vi "saveImage.vi"(8 "error in (no error)":errorcluster, 9 "16bit image data":i16[][](array[numeric]), 10 "Path":path, 11 "Pixelfly in":refnum<class "Pixelfly.lvclass">) -> (0 "error out":errorcluster, 3 "Pixelfly out":refnum<class "Pixelfly.lvclass">)   [LabVIEW 2009]
uses:
  Camera/Camera.lvclass
  Camera/Pixelfly/Pixelfly.lvclass
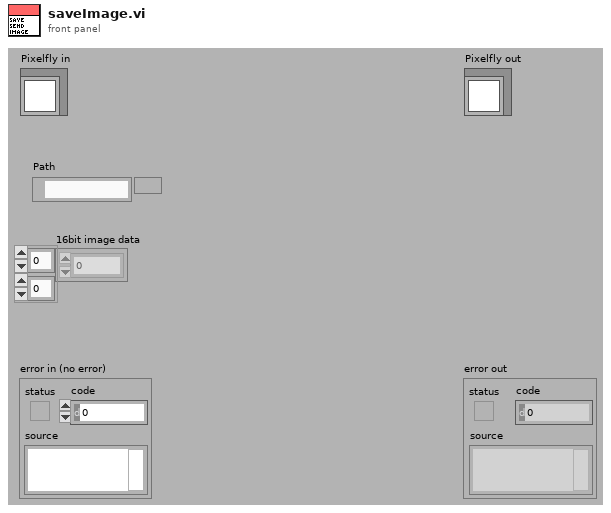
[diagram p1: front panel]
types:
  T1 = typedef "Image Type" = u32
  T2 = typedef "IMAQ Image.ctl" = refnum<image>
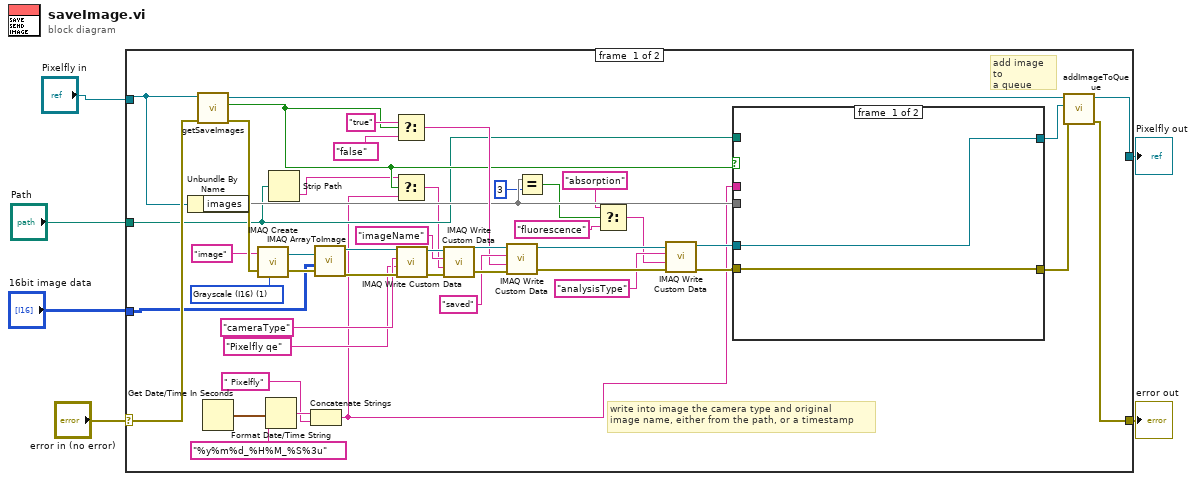
[diagram p0: block diagram]
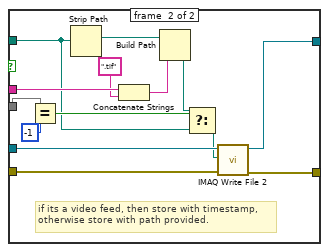
[diagram p2: hidden frame]
diagram:
  n1 = case shown="No Error" "error in (no error)" {
    selector: "error in (no error)" -> [w52 w70]
    tunnel: [w44 w70] -> w5
    tunnel: [w45 w69] -> w3
    tunnel: "Pixelfly in" -> [w25 w69]
    tunnel: "Path" -> [w11 _]
    tunnel: "16bit image data" -> [w7 _]
    frame #0 {
      w49 = T1 1 items=["Grayscale (U8)", "Grayscale (I16)", "Grayscale (SGL)", "Complex (CSG)", "RGB (U32)", "HSL (U32)", "RGB (U64)", "Grayscale (U16)"] ("Image Type")
      # "write into image the camera type and original\nimage name, either from the path, or a timestamp"
      # "add image to\na queue"
      n2 = Unbundle By Name(w25) -> ("images"=w21)
      n3 = call "getSaveImages.vi"("error in (no error)"=w52, "Camera in"=w25) -> ("error out"=w51:errorcluster, "saveImages?"=w12:bool, "Camera out"=w46:refnum<class "Pixelfly.lvclass">)  [unwired: 7 in]
      n4 = Get Date/Time In Seconds() -> (seconds since 1Jan1904=w39:timestamp)
      n5 = call "IMAQ Create"("Image Name"="image", "Image Type"=w49, "error in (no error)"=w51) -> ("New Image"=w48:T2, "error out"=w47:errorcluster)  [unwired: 2 in]
      n6 = Format Date/Time String(time format string (%c)="%y%m%d_%H%M_%S%3u", seconds (now)=w39) -> (date/time string=w37:string)  [unwired: 1 in]
      n7 = Strip Path(path=w11) -> (name=w10:string)  [unwired: 1 out]
      n8 = Concatenate Strings(w37, " Pixelfly") -> (w9:string)
      n9 = call "IMAQ ArrayToImage"("error in (no error)"=w47, "Image Pixels (I16)"=w7, "Image"=w48) -> ("error out"=w42:errorcluster, "Image Out"=w43:T2)  [unwired: 7 in]
      n10 = Select(t="true", s=w12, f="false") -> (s? t:f=w28:string)
      n11 = Select(t=w10, s=w12, f=w9) -> (s? t:f=w8:string)
      n12 = call "IMAQ Write Custom Data"("error in (no error)"=w42, "Custom Data In"="Pixelfly qe", "Key"="cameraType", "Image"=w43) -> ("error out"=w35:errorcluster, "Image Out"=w34:T2)  [unwired: 6 in]
      n13 = call "IMAQ Write Custom Data"("error in (no error)"=w35, "Custom Data In"=w8, "Key"="imageName", "Image"=w34) -> ("error out"=w33:errorcluster, "Image Out"=w32:T2)  [unwired: 6 in]
      n14 = call "IMAQ Write Custom Data"("error in (no error)"=w33, "Custom Data In"=w28, "Key"="saved", "Image"=w32) -> ("error out"=w23:errorcluster, "Image Out"=w24:T2)  [unwired: 6 in]
      n15 = Equal?(x=w21, y=3) -> (x = y?=w19:bool)
      n16 = Select(t="absorption", s=w19, f="fluorescence") -> (s? t:f=w16:string)
      n17 = call "IMAQ Write Custom Data"("error in (no error)"=w23, "Custom Data In"=w16, "Key"="analysisType", "Image"=w24) -> ("error out"=w14:errorcluster, "Image Out"=w15:T2)  [unwired: 6 in]
      n18 = case shown="True" w12 {
        tunnel: w14 -> [w53 w68]
        tunnel: [w53 w67] -> w26
        tunnel: w15 -> [w54 w66]
        tunnel: [w54 w65] -> w27
        tunnel: w11 -> [_ w56]
        tunnel: w9 -> [_ w63]
        tunnel: w21 -> [_ w60]
        frame #0 {
        }
        frame #1 {
          # "if its a video feed, then store with timestamp,\notherwise store with path provided."
          n19 = Equal?(x=w60, y=-1) -> (x = y?=w57:bool)
          n20 = Strip Path(path=w56) -> (stripped path=w64:path)  [unwired: 1 out]
          n21 = Concatenate Strings(w63, ".tif") -> (w61:string)
          n22 = Build Path(base path=w64, name or relative path=w61) -> (appended path=w58:path)
          n23 = Select(t=w58, s=w57, f=w56) -> (s? t:f=w55:path)
          n24 = call-poly "IMAQ Write File 2"("error in (no error)"=w68, "File Path"=w55, "Image"=w66) -> ("error out"=w67:errorcluster, "Image Out (duplicate)"=w65:T2)  [unwired: 7 in]
        }
      }
      n25 = call "addImageToQueue.vi"("error in (no error)"=w26, "Image"=w27, "Camera in"=w46) -> ("error out"=w44:errorcluster, "Camera out"=w45:refnum<class "Pixelfly.lvclass">)  [unwired: 7 in]
    }
    frame #1 {
    }
  }
  "error out" <- w5
  "Pixelfly out" <- w3
